vi "Stop Core.vi"(10 "final error code":i32, 11 "Nested in":refnum<class "Controller.lvclass">) -> (3 "Nested out":refnum<class "Controller.lvclass">)   [LabVIEW 2020, in "Controller.lvlib" / "Controller.lvclass"]
doc: "(<B>Filename</B>: Actor Framework.lvlib:Actor.lvclass:Stop Core.vi)\n\nDefines what the actor does before it stops. Use the <B>final error code</B> input to determine whether the actor shut down in response to an error.\n\nBy default, this method does nothing. A descendant class may override it to define behavior, such as shutting down any processes the actor initiated in its override of the Actor Core method."
uses:
  Controller.lvclass
  <vilib>/ActorFramework/Actor/Actor.lvclass
  Controller.lvclass/Controller.ctl
  <vilib>/ActorFramework/Stop Msg/Stop Msg.lvclass
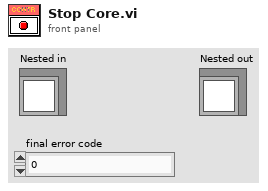
[diagram p1: front panel]
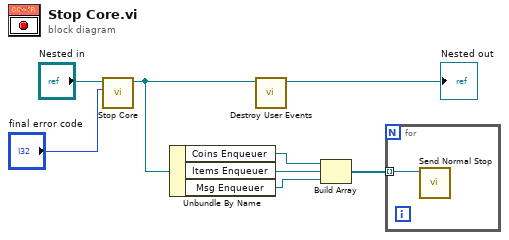
[diagram p0: block diagram]
diagram:
  n1 = call-parent "Stop Core.vi"("final error code"="final error code", "Actor in"="Nested in") -> ("Actor out"=w5:refnum<class "Controller.lvclass">)  [unwired: 9 in]
  n2 = Unbundle By Name(w5) -> ("Coins Enqueuer"=w4:refnum<class "Message Enqueuer.lvclass">, "Items Enqueuer"=w3:refnum<class "Message Enqueuer.lvclass">, "Msg Enqueuer"=w2:refnum<class "Message Enqueuer.lvclass">)
  n3 = call "Destroy User Events.vi"("UI Template in"=w5) -> ("UI Template out"=→"Nested out":refnum<class "Controller.lvclass">)  [unwired: 10 in]
  n4 = Build Array(w4, w3, w2) -> (w1:refnum<class "Message Enqueuer.lvclass">[])
  n5 = for {
    tunnel: w1 -> [w9] mode=indexing
    n6 = call <vilib>:"Send Normal Stop.vi"("Message Enqueuer"=w9) -> ()  [unwired: 10 in, 1 out]
  }
